vi "gen.vi"() -> ()   [LabVIEW 2013]
uses:
  <vilib>/sound2/lvsound2.llb/Sound Data Format.ctl
  <vilib>/sound2/lvsound2.llb/Sampling Mode.ctl
  <vilib>/sound2/lvsound2.llb/Sound Input Read (DBL).vi
  <vilib>/sound2/lvsound2.llb/Sound Output Set Volume (Single).vi
  <vilib>/sound2/lvsound2.llb/Sound Output Write (DBL Single).vi
panel:
  in  "milliseconds to wait":u32(knob) scale=0.0..1000.0
  out "Generated Sound 2":waveform(dbl)(graph)
  in  "Input Device ID":u32
  in  "Phase":dbl(knob) scale=0.0..10.0
  out "Numeric":dbl
  out "Hz":dbl
  out "Y min":dbl format="%0.2f"
  out "Y max":dbl format="%0.2f"
  in  "Device ID":u32
  in  "Stop":bool
  in  "Frequency":dbl(knob)=500.0 scale=0.0..10000.0
  out "Generated Sound":waveform(dbl)(graph)
  in  "Volume":dbl(knob)=50.0 scale=0.0..100.0
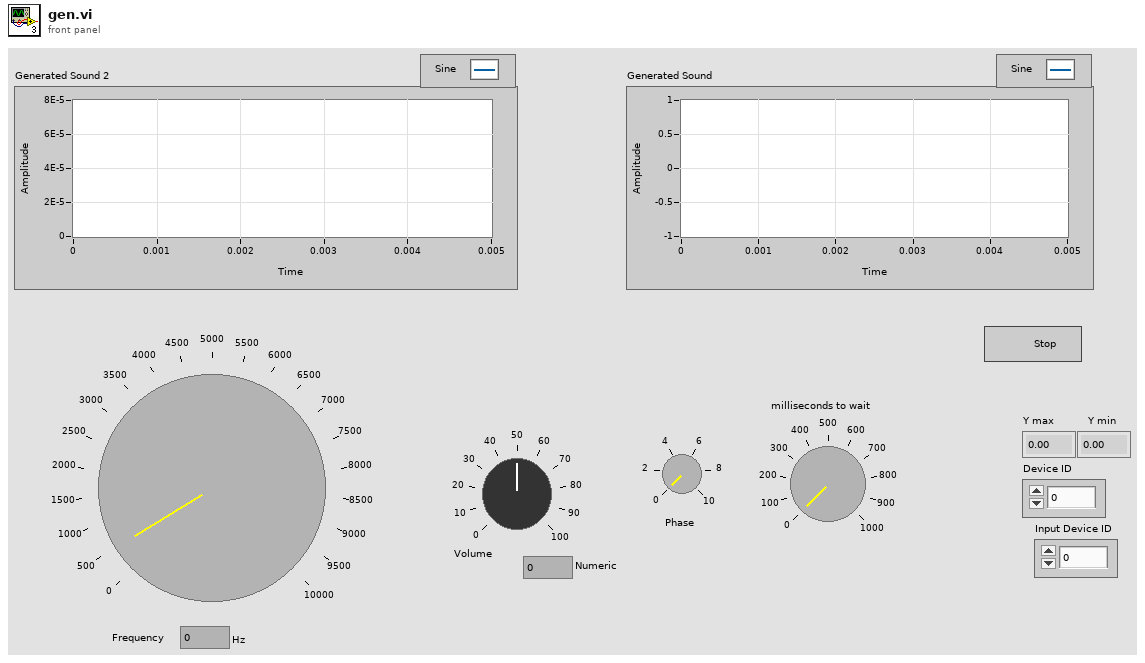
[diagram p1: front panel]
types:
  T1 = typedef "Sound Data Format.ctl" = cluster{"sample rate (S/s)":dbl, "number of channels":i32, "bits per sample":i32}
  T2 = typedef "Sampling Mode.ctl" = i32
  T3 = typedef "Sound Output Task ID.ctl" = u32
  T4 = typedef "Sound Input Task ID.ctl" = u32
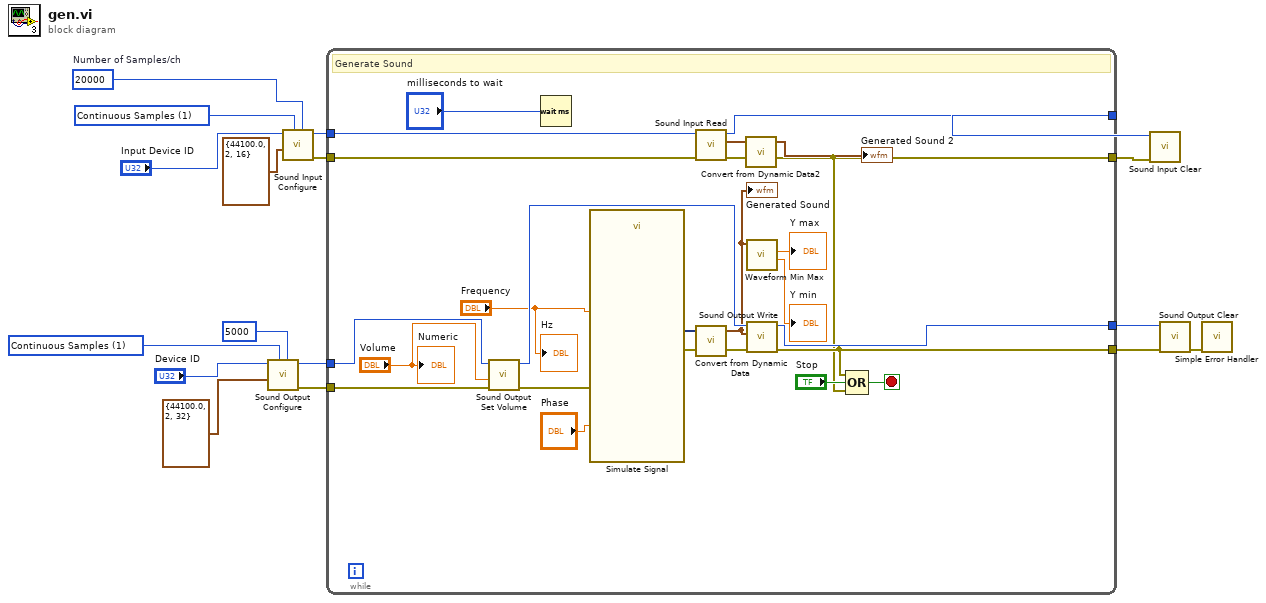
[diagram p0: block diagram]
diagram:
  w5 = 20000  # Number of Samples/ch
  w7 = T2 1 items=["Finite Samples", "Continuous Samples"] ("sample mode")
  w12 = T2 1 items=["Finite Samples", "Continuous Samples"] ("sample mode")
  n1 = call <vilib>:"Sound Output Configure.vi"("number of samples/ch"=5000 ("Number of Samples/ch"), "sample mode"=w12, "sound format"=T1 {"sample rate (S/s)"=44100.0, "number of channels"=2, "bits per sample"=32} ("Sound Format"), "device ID"="Device ID") -> ("error out"=w17:errorcluster, "task ID"=w16:T3)  [unwired: 6 in]
  n2 = call <vilib>:"Sound Input Configure.vi"("number of samples/ch"=w5, "sample mode"=w7, "sound format"=T1 {"sample rate (S/s)"=44100.0, "number of channels"=2, "bits per sample"=16} ("Sound Format"), "device ID"="Input Device ID") -> ("error out"=w1:errorcluster, "task ID"=w4:T4)  [unwired: 6 in]
  n3 = while {
    tunnel: w16 -> [w37]
    tunnel: [w40] -> w14
    tunnel: w17 -> [w39]
    tunnel: [w22] -> w15
    tunnel: w4 -> [w27]
    tunnel: [w20] -> w3
    tunnel: [w26] -> w2
    tunnel: w1 -> [w18]
    stop <- w19 stop-if-true
    # "Generate Sound"
    n4 = call-poly <vilib>:"Sound Output Set Volume.vi"("error in (no error)"=w39, "volume"="Volume", "task ID"=w37) -> ("error out"=w36:errorcluster, "task ID out"=w38:T3)  [unwired: 7 in]
    n5 = Wait (ms)(milliseconds to wait="milliseconds to wait") -> ()  [unwired: 1 out]
    n6 = call "Simulate Signal"("Frequency"="Frequency", "Phase"="Phase", "error in (no error)"=w36) -> ("Sine"=w34:dynamicdata, "error out"=w35:errorcluster)  [unwired: 11 in]
    n7 = call-poly <vilib>:"Sound Input Read.vi"("error in (no error)"=w18, "task ID"=w27) -> ("error out"=w20:errorcluster, "data"=w25:waveform(dbl)[], "task ID out"=w26:T4)  [unwired: 7 in]
    n8 = call "Convert from Dynamic Data"("Dynamic Data Type"=w34) -> ("Waveform"=w28:waveform(dbl))  [unwired: 3 in]
    "Generated Sound" <- w28
    n9 = call "Convert from Dynamic Data2"("Dynamic Data Type"=w25) -> ("Waveform"=→"Generated Sound 2":waveform(dbl))  [unwired: 3 in]
    n10 = call <vilib>:"Waveform Min Max.vi"("waveform in"=w28) -> ("Y min"=→"Y min":dbl, "Y max"=→"Y max":dbl)  [unwired: 5 in, 4 out]
    n11 = call-poly <vilib>:"Sound Output Write.vi"("error in (no error)"=w35, "data"=w28, "task ID"=w38) -> ("error out"=w22:errorcluster, "task ID out"=w40:T3)  [unwired: 7 in]
    n12 = Compound Arithmetic op=OR(w22, "Stop", w20) -> (w19:bool)
    "Hz" <- "Frequency"
    "Numeric" <- "Volume"
  }
  n13 = call <vilib>:"Sound Input Clear.vi"("error in (no error)"=w3, "task ID"=w2) -> ()  [unwired: 9 in, 1 out]
  n14 = call <vilib>:"Sound Output Clear.vi"("error in (no error)"=w15, "task ID"=w14) -> ("error out"=w10:errorcluster)  [unwired: 9 in]
  n15 = call <vilib>:"Simple Error Handler.vi"("error in (no error)"=w10) -> ()  [unwired: 4 in, 5 out]
